vi "VerifAllChanDiscon.vi"(8 "error in (no error)":errorcluster, 11 "S4GUI in":refnum<class "S4GUI.lvclass">) -> (0 "error out":errorcluster, 2 "All disconnected":bool, 3 "S4GUI out":refnum<class "S4GUI.lvclass">)   [LabVIEW 2018, in "S4GUI.lvclass"]
uses:
  S4GUI.lvclass
  S4GUI.lvclass/S4GUI.ctl
  Server/Server.lvclass/Server.ctl
  Acquisition/Acquisition.lvclass
  C:/Users/devstaff/sparc4/s4gui/Versao ZeroMQ REQ-REP/SPARC4_GUI -v1.0.8 - reconhecimento do ACK do ACS/Server/Server.lvclass
  Server/Server.lvclass
panel:
  # "F: At least one channel connected\nT: All channels disconnected"
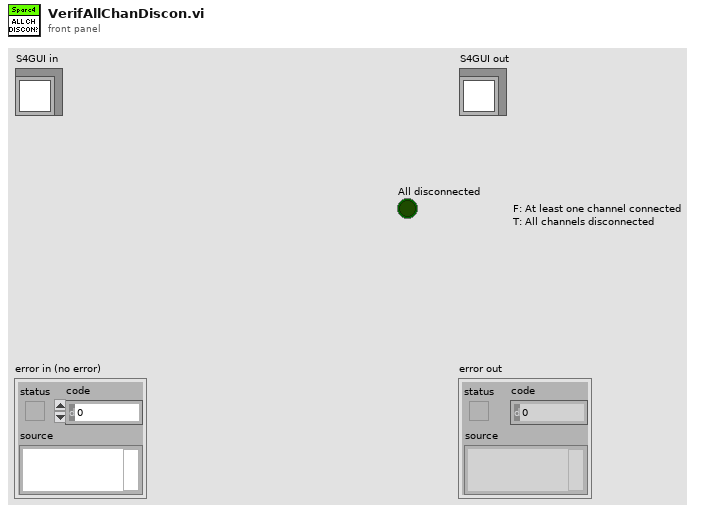
[diagram p1: front panel]
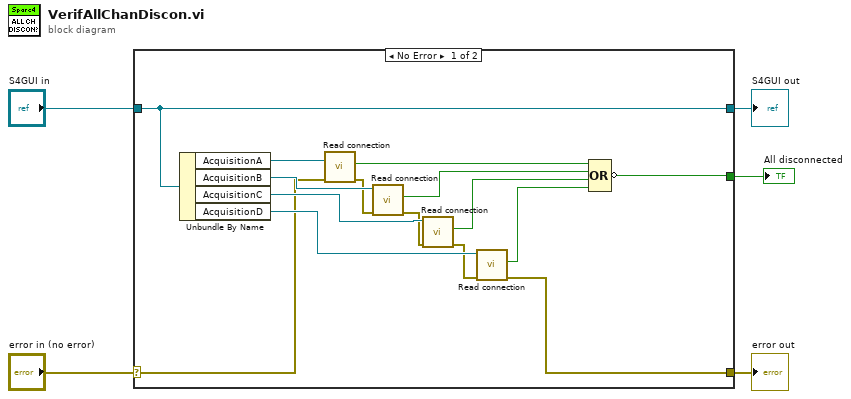
[diagram p0: block diagram]
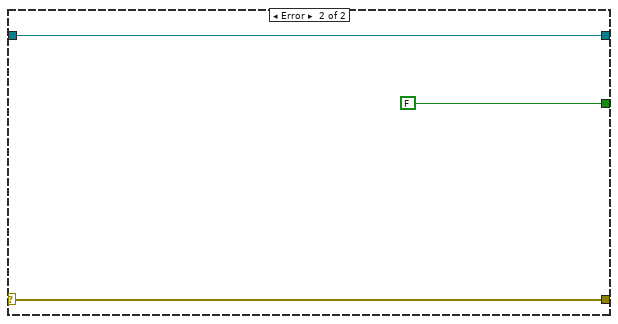
[diagram p2: hidden frame]
diagram:
  n1 = case shown="No Error" "error in (no error)" {
    selector: "error in (no error)" -> [w15 w23]
    tunnel: [w6 w23] -> w4
    tunnel: [w20 w22] -> w2
    tunnel: "S4GUI in" -> [w20 w22]
    tunnel: [w7 FALSE] -> w1
    frame No Error {
      n2 = Unbundle By Name(w20) -> ("AcquisitionA"=w19:refnum<class "Acquisition.lvclass">, "AcquisitionB"=w18:refnum<class "Acquisition.lvclass">, "AcquisitionC"=w17:refnum<class "Acquisition.lvclass">, "AcquisitionD"=w16:refnum<class "Acquisition.lvclass">)
      n3 = call "Read connection.vi"("error in (no error)"=w15, "Server in"=w19) -> ("error out"=w14:errorcluster, "connection"=w11:bool)  [unwired: 7 in, 1 out]
      n4 = call "Read connection.vi"("error in (no error)"=w14, "Server in"=w18) -> ("error out"=w13:errorcluster, "connection"=w10:bool)  [unwired: 7 in, 1 out]
      n5 = call "Read connection.vi"("error in (no error)"=w13, "Server in"=w17) -> ("error out"=w12:errorcluster, "connection"=w9:bool)  [unwired: 7 in, 1 out]
      n6 = call "Read connection.vi"("error in (no error)"=w12, "Server in"=w16) -> ("error out"=w6:errorcluster, "connection"=w8:bool)  [unwired: 7 in, 1 out]
      n7 = Compound Arithmetic op=OR(w11, w10, w9, w8) -> (invert w7:bool)
    }
    frame Error {
    }
  }
  "error out" <- w4
  "S4GUI out" <- w2
  "All disconnected" <- w1
